vi "Class Method Property File Paths.vi"(8 "error in (no error)":errorcluster) -> (0 "error out":errorcluster, 1 "Method Ini":path, 2 "Property Ini":path, 3 "Class Ini":path)   [LabVIEW 2023]
doc: "Return paths to class/property/methods xml support files based on the current LV version"
panel:
  # "C:\\Users\\drwag\\Documents\\LabVIEW\\BundleMagic\\Source Code\\Source Code Support"
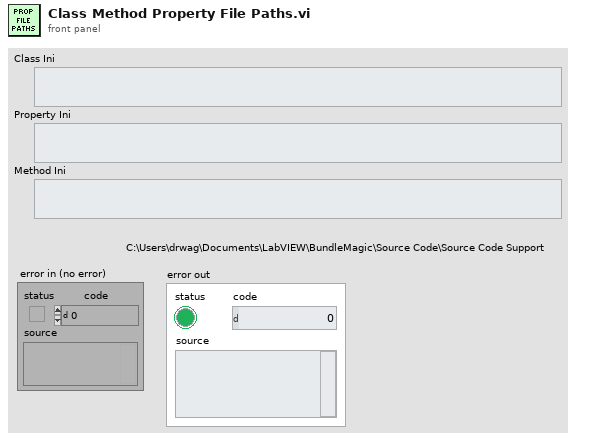
[diagram p1: front panel]
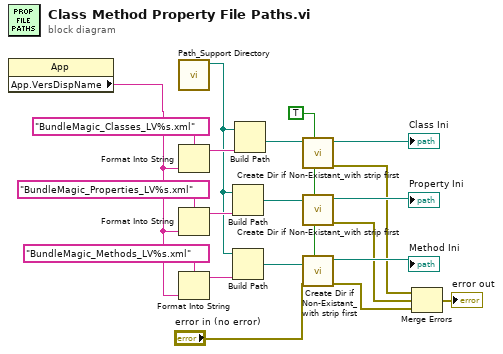
[diagram p0: block diagram]
diagram:
  w7 = TRUE ("Strip Path First [F]")
  n1 = property class="App"() -> ("App.VersDispName"=w20:string)  [unwired: 2 in, 2 out]
  n2 = call "Path_Support Directory.vi"() -> ("Support Directory"=w1:path)  [unwired: 11 in]
  n3 = Format Into String(format string="BundleMagic_Classes_LV%s.xml", w20) -> (resulting string=w15:string)  [unwired: 2 in, 1 out]
  n4 = Format Into String(format string="BundleMagic_Properties_LV%s.xml", w20) -> (resulting string=w16:string)  [unwired: 2 in, 1 out]
  n5 = Format Into String(format string="BundleMagic_Methods_LV%s.xml", w20) -> (resulting string=w19:string)  [unwired: 2 in, 1 out]
  n6 = Build Path(base path=w1, name or relative path=w16) -> (appended path=w12:path)
  n7 = Build Path(base path=w1, name or relative path=w19) -> (appended path=w11:path)
  n8 = Build Path(base path=w1, name or relative path=w15) -> (appended path=w13:path)
  n9 = call "Create Dir if Non-Existant_with strip first.vi"("Strip Path First [F]"=w7, "Directory Path"=w13) -> ("error out"=w6:errorcluster, "dup Directory Path"=→"Class Ini":path)  [unwired: 7 in, 1 out]
  n10 = call "Create Dir if Non-Existant_with strip first.vi"("Strip Path First [F]"=w7, "Directory Path"=w12) -> ("error out"=w5:errorcluster, "dup Directory Path"=→"Property Ini":path)  [unwired: 7 in, 1 out]
  n11 = call "Create Dir if Non-Existant_with strip first.vi"("Strip Path First [F]"=w7, "error in (no error)"="error in (no error)", "Directory Path"=w11) -> ("error out"=w4:errorcluster, "dup Directory Path"=→"Method Ini":path)  [unwired: 6 in, 1 out]
  n12 = Merge Errors(w6, w5, w4) -> (→"error out":errorcluster)
